vi "Inspect.vi"(8 "error in (no error)":errorcluster, 11 "Message in":refnum<class "Message.lvclass">) -> (0 "error out":errorcluster, 1 "Data":variant, 2 "Name":string, 3 "Message out":refnum<class "Message.lvclass">, 5 "Reply Channel":refnum<notifier>)   [LabVIEW 2015, in "Message.lvclass"]
uses:
  Message.lvclass
  Message.lvclass/Message.ctl
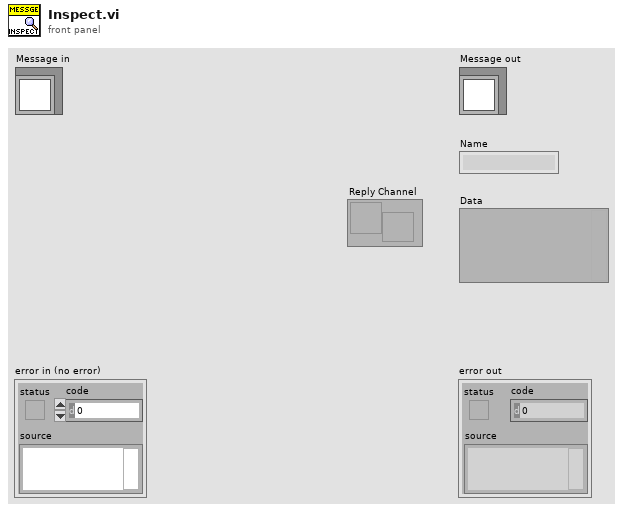
[diagram p1: front panel]
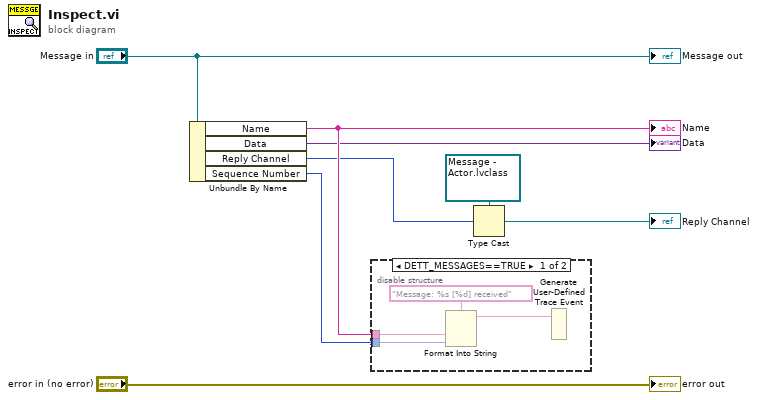
[diagram p0: block diagram]
diagram:
  n1 = Unbundle By Name("Message in") -> ("Name"=w6:string, "Data"=→"Data":variant, "Reply Channel"=w3:u32, "Sequence Number"=w4:u64)
  "Name" <- w6
  n2 = disable-structure shown="DETT_MESSAGES==TRUE" {
    disable-tunnel: w6 -> [w10 _]
    disable-tunnel: w4 -> [w9 _]
    frame condition #0 {
      n3 = Format Into String(format string="Message: %s [%d] received", w10, w9) -> (resulting string=w11:string)  [unwired: 2 in, 1 out]
      n4 = Generate User-Defined Trace Event(2:w11) -> ()  [unwired: 1 in]
    }
    frame condition #1 (active) {
    }
  }
  n5 = Type Cast(type=refnum<notifier> refnum ("Reply Channel"), x=w3) -> (*(type *) &x=→"Reply Channel":refnum<notifier>)
  "error out" <- "error in (no error)"
  "Message out" <- "Message in"
